vi "Set travel parameters.vi"(8 "Error In":errorcluster, 9 "Motor settings array":T1[](array[typedef]) {"N cycles" step=1; "IM Idle time" format="%.0fms"; "Travel distance" format="%#_gmm"; "Speed" format="%#_gmm/s"}, 11 "VISA resource in":refnum<visa-resource-name>) -> (0 "Error Out":errorcluster, 3 "VISA resource out":refnum<visa-resource-name>)   [LabVIEW 2014, in "Motor manager.lvlib"]
uses:
  Motor manager.lvlib
  Typedef/Motor settings.ctl
  Typedef/Motor.ctl
  Typedef/Move type.ctl
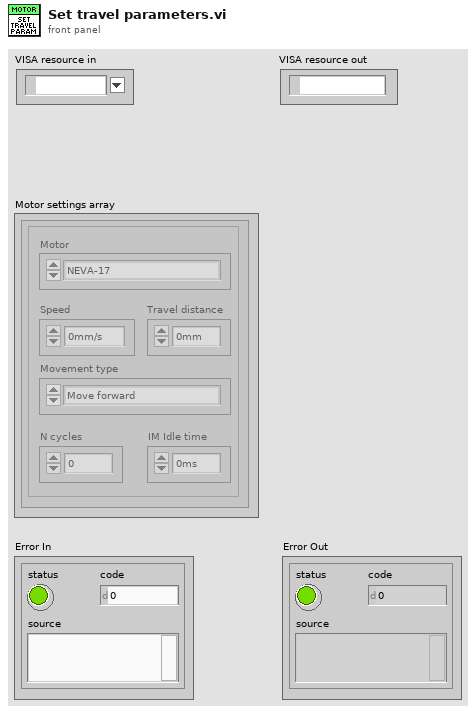
[diagram p1: front panel]
types:
  T1 = typedef "Motor manager.lvlib/Motor settings.ctl" = cluster{"Motor":T2, "Speed":sgl, "Travel distance":sgl, "Movement type":T3, "IM Idle time":u32, "N cycles":u32}
  T2 = typedef "Motor manager.lvlib/Motor.ctl" = enum16{"NEVA-17"}
  T3 = typedef "Motor manager.lvlib/Move type.ctl" = enum16{"Move forward", "Move backward", "Cycle (forward first)", "Cycle (backward first)"}
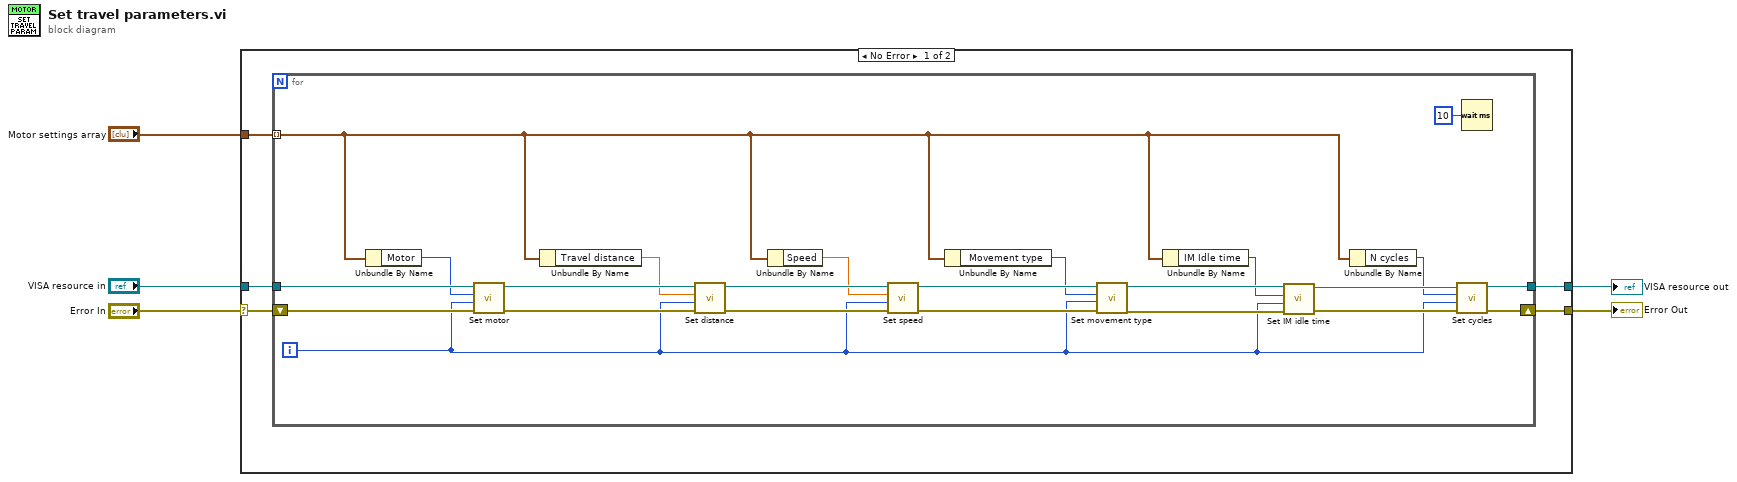
[diagram p0: block diagram]
diagram:
  n1 = case shown="No Error" "Error In" {
    selector: "Error In" -> [w10 w35]
    tunnel: [w9 w35] -> w4
    tunnel: "VISA resource in" -> [w8 w34]
    tunnel: [w7 w34] -> w2
    tunnel: "Motor settings array" -> [w6 _]
    frame No Error {
      n2 = for {
        tunnel: w6 -> [w19] mode=indexing
        shift-right: [w29] -> w9
        shift-left: w10 -> [w33]
        tunnel: w8 -> [w28]
        tunnel: [w24] -> w7
        i -> [w11]
        n3 = Unbundle By Name(w19) -> ("Motor"=w16:T2)
        n4 = call "Set motor.vi"("Error In"=w33, "Motor index"=w11, "Motor"=w16, "VISA resource in"=w28) -> ("Error Out"=w32:errorcluster, "VISA resource out"=w27:refnum<visa-resource-name>)  [unwired: 6 in]
        n5 = Unbundle By Name(w19) -> ("Travel distance"=w17:sgl)
        n6 = call "Set distance.vi"("Error In"=w32, "Motor index"=w11, "Travel distance"=w17, "VISA resource in"=w27) -> ("Error Out"=w31:errorcluster, "VISA resource out"=w26:refnum<visa-resource-name>)  [unwired: 6 in]
        n7 = Unbundle By Name(w19) -> ("Speed"=w13:sgl)
        n8 = call "Set speed.vi"("Error In"=w31, "Motor index"=w11, "Speed"=w13, "VISA resource in"=w26) -> ("Error Out"=w30:errorcluster, "VISA resource out"=w25:refnum<visa-resource-name>)  [unwired: 6 in]
        n9 = Unbundle By Name(w19) -> ("Movement type"=w14:T3)
        n10 = call "Set movement type.vi"("Error In"=w30, "Motor index"=w11, "Movement type"=w14, "VISA resource in"=w25) -> ("Error Out"=w20:errorcluster, "VISA resource out"=w23:refnum<visa-resource-name>)  [unwired: 6 in]
        n11 = Unbundle By Name(w19) -> ("IM Idle time"=w15:u32)
        n12 = call "Set IM idle time.vi"("Error In"=w20, "Motor index"=w11, "IM Idle time"=w15, "VISA resource in"=w23) -> ("Error Out"=w21:errorcluster, "VISA resource out"=w22:refnum<visa-resource-name>)  [unwired: 6 in]
        n13 = Unbundle By Name(w19) -> ("N cycles"=w12:u32)
        n14 = call "Set cycles.vi"("Error In"=w21, "Motor index"=w11, "N cycles"=w12, "VISA resource in"=w22) -> ("Error Out"=w29:errorcluster, "VISA resource out"=w24:refnum<visa-resource-name>)  [unwired: 6 in]
        n15 = Wait (ms)(milliseconds to wait=u32 10) -> ()  [unwired: 1 out]
      }
    }
    frame Error {
    }
  }
  "VISA resource out" <- w2
  "Error Out" <- w4
